vi "FlatToRichni_measurementlink_measurement_v2_MeasureResponse.vi"(5 "OutputClusterType":T1, 11 "InputCluster":T3) -> (3 "OutputCluster":T1)   [LabVIEW 2020, in "Measurement Service Client V2.lvlib"]
uses:
  Measurement Service Client V2.lvlib
  ni_measurementlink_measurement_v2_MeasureResponse_Flat.ctl
  google_protobuf_Any_Flat.ctl
  ni_measurementlink_measurement_v2_MeasureResponse.ctl
  google_protobuf_Any.ctl
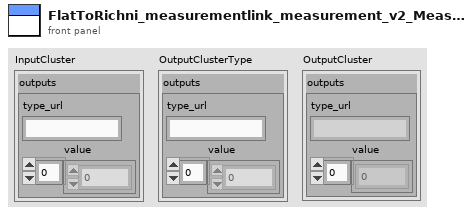
[diagram p1: front panel]
types:
  T1 = typedef "Measurement Service Client V2.lvlib/ni_measurementlink_measurement_v2_MeasureResponse.ctl" = cluster{"outputs":T2}
  T2 = typedef "Measurement Service Client V2.lvlib/google_protobuf_Any.ctl" = cluster{"type_url":string, "value":u8[]}
  T3 = typedef "Measurement Service Client V2.lvlib/ni_measurementlink_measurement_v2_MeasureResponse_Flat.ctl" = cluster{"outputs":T4}
  T4 = typedef "Measurement Service Client V2.lvlib/google_protobuf_Any_Flat.ctl" = cluster{"type_url":string, "value":u8[]}
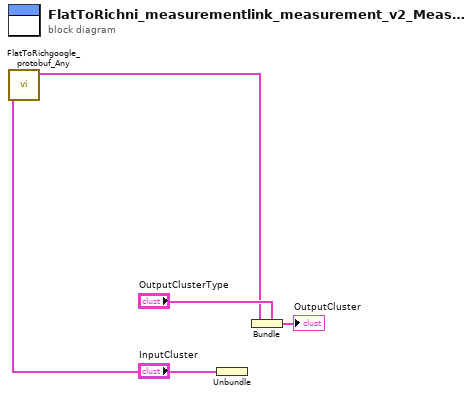
[diagram p0: block diagram]
diagram:
  n1 = Unbundle "Unbundle"("InputCluster") -> ("outputs"=w2:T4)
  n2 = call "FlatToRichgoogle_protobuf_Any.vi"("InputCluster"=w2) -> ("OutputCluster"=w1:T2)  [unwired: 10 in]
  n3 = Bundle "Bundle"(cluster="OutputClusterType", "outputs"=w1) -> (→"OutputCluster":T1)
